vi "ReadObjectLayout.vi"(7 "properties to ignore":variant, 8 "error in (no error)":errorcluster, 10 "GObj Refnum":refnum<vi>, 11 "Path Control Layout in":refnum<class "Path Control Layout.lvclass">) -> (0 "error out":errorcluster, 3 "Path Control Layout out":refnum<class "Path Control Layout.lvclass">)   [LabVIEW 2012, in "NI_SE_Front Panel Layout.lvlib" / "Path Control Layout.lvclass"]
doc: "Read layout information from the GObj Refnum."
uses:
  Path Control Layout.lvclass
  Control Layout/Control Layout.lvclass
  Path Control Layout.lvclass/Path Control Layout.ctl
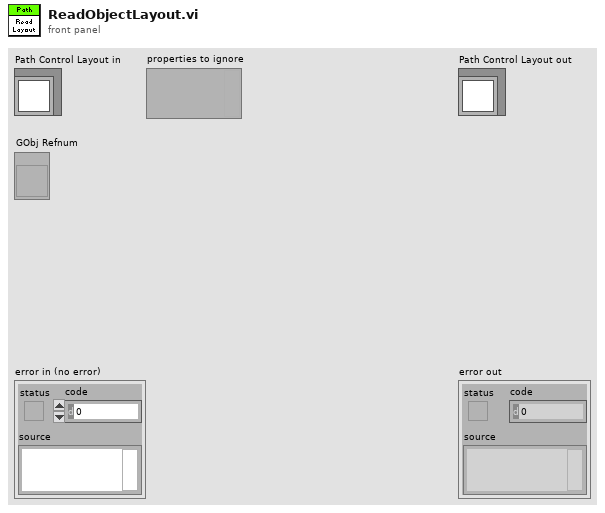
[diagram p1: front panel]
types:
  T1 = typedef "LVFontTypeDef.ctl" = cluster{"Font Name":string, "Size":u16, "Bold":bool, "Italic":bool, "Underline":bool, "Strikeout":bool, "Color":u32}
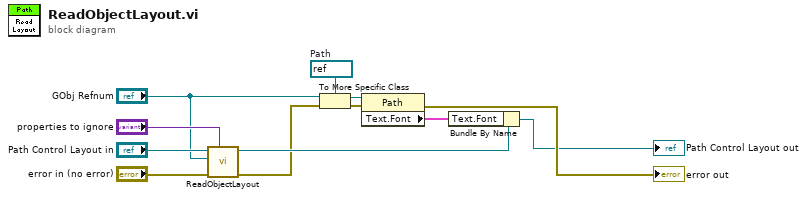
[diagram p0: block diagram]
diagram:
  w9 = refnum<vi> refnum  # Path
  n1 = call-parent "ReadObjectLayout.vi"("properties to ignore"="properties to ignore", "error in (no error)"="error in (no error)", "GObj Refnum"="GObj Refnum", "Control Layout in"="Path Control Layout in") -> ("error out"=w4:errorcluster, "Control Layout out"=w5:refnum<class "Path Control Layout.lvclass">)  [unwired: 6 in]
  n2 = To More Specific Class(target class=w9, reference="GObj Refnum", error in=w4) -> (specific class reference=w8:refnum<vi>, error out=w7:errorcluster)
  n3 = property class="Path"(reference=w8, error in=w7) -> (error out=→"error out":errorcluster, "Text.Font"=w6:T1)  [unwired: 1 out]
  n4 = Bundle By Name(cluster=w5, "Text.Font"=w6) -> (→"Path Control Layout out":refnum<class "Path Control Layout.lvclass">)
